vi "Autonomous Independent.vi"() -> ()   [LabVIEW 2012]
doc: "This VI is called when autonomous begins, and will automatically be terminated when autonomous ends. You can carry out timed or sensor driven robot movement independently without needing to return to the caller."
uses:
  <vilib>/Rock Robotics/WPI/Solenoid/WPI_SolenoidValue.ctl
  Robot Global Data.vi
  <vilib>/Rock Robotics/WPI/Compressor/WPI_CompressorGetSetRefNum.vi
  <vilib>/Rock Robotics/WPI/RobotDrive/WPI_RobotDriveGetSetRefNum.vi
  <vilib>/Rock Robotics/WPI/Solenoid/WPI_SolenoidSetEnum.vi
  <vilib>/Rock Robotics/WPI/RobotDrive/WPI_RobotDriveArcadeDrive_Standard(NoSaturation).vi
panel:
  out "Current Movement, for debugging":T1 {"Y Joystick Value" scale=1.0..-1.0; "X Joystick Value" scale=-1.0..1.0}
  in  "Array of robot movements":T2(array[cluster]) {"Y Joystick Value" scale=1.0..-1.0; "X Joystick Value" scale=-1.0..1.0}
  # "Be sure to right-click and choose Data Operations>>Make Current Value default if you want to save the array values with the VI"
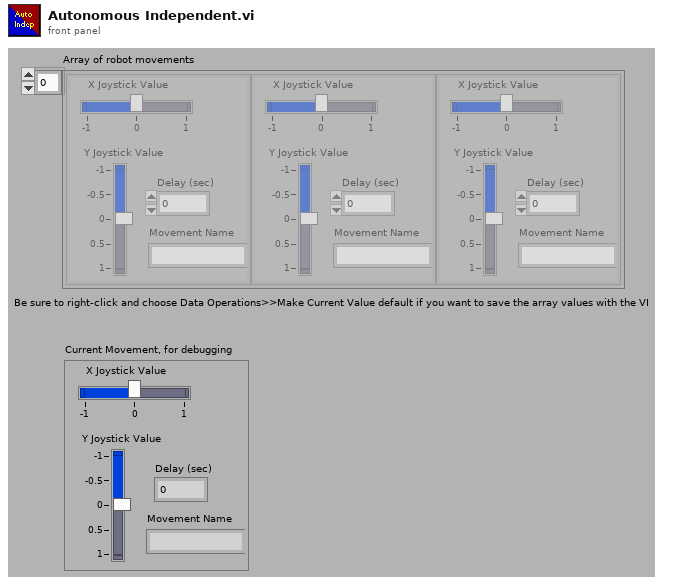
[diagram p1: front panel]
types:
  T1 = cluster{"X Joystick Value":dbl, "Y Joystick Value":dbl, "Delay (sec)":dbl, "Movement Name":string}
  T2 = cluster{"X Joystick Value":dbl, "Y Joystick Value":dbl, "Delay (sec)":dbl, "Movement Name":string}[]
  T3 = typedef "WPI_SolenoidDevRef.ctl" = cluster{"DevStatus":errorcluster, "Solenoid Module":T4, "Forward Solenoid Channel":T5, "Reverse Solenoid Channel":T5}
  T4 = typedef "FPGA_TypedefSolenoidModule.ctl" = enum16{"Solenoid Module 1", "Solenoid Module 2"}
  T5 = typedef "WPI_SolenoidChannel.ctl" = enum8{"Solenoid 1", "Solenoid 2", "Solenoid 3", "Solenoid 4", "Solenoid 5", "Solenoid 6", "Solenoid 7", "Solenoid 8", "Invalid"}
  T6 = typedef "WPI_MotorControlDeviceRef.ctl" = cluster{"DeviceStatus":errorcluster, "Type":enum16{"PWM", "CAN"}, "PWM":cluster{"Digital Module":T7, "PWM Channel":T8, "DeadBand":T9}, "CAN":cluster{"Device Number":u8, "Control Mode":T10, "Semaphore":T11, "Max Vout":dbl}, "Invert":bool, "TransformRef":T12, "InvTransformRef":T12}
  T7 = typedef "FPGA_TypedefDigitalModule.ctl" = enum16{"Digital Module 1", "Digital Module 2"}
  T8 = typedef "FPGA_DIOPWMChannel.ctl" = enum8{"PWM 1", "PWM 2", "PWM 3", "PWM 4", "PWM 5", "PWM 6", "PWM 7", "PWM 8", "PWM 9", "PWM 10", "Invalid"}
  T9 = typedef "WPI_PWMDeadband.ctl" = cluster{"Name":string, "maxPositivePwm":i32, "minPositivePwm":i32, "centerPwm":i32, "maxNegativePwm":i32, "minNegativePwm":i32, "angularRange":u16}
  T10 = typedef "WPI_CANJaguar_ControlMode.ctl" = enum8{"Percent VBus", "Current", "Speed", "Position", "Voltage"}
  T11 = typedef "Semaphore RefNum" = refnum<k1>
  T12 = typedef "WPI_PWMTransform_ConPane.ctl" = refnum<vi>
  T13 = typedef "WPI_DigitalInputDevRef.ctl" = cluster{"DevStatus":errorcluster, "DIO Channel":T14, "Digital Module":T7}
  T14 = typedef "FPGA_DIOChannel.ctl" = enum8{"DIO 1", "DIO 2", "DIO 3", "DIO 4", "DIO 5", "DIO 6", "DIO 7", "DIO 8", "DIO 9", "DIO 10", "DIO 11", "DIO 12", "DIO 13", "DIO 14", "Invalid"}
  T15 = typedef "WPI_SolenoidValue.ctl" = enum16{"Off", "On", "Forward", "Reverse"}
  T16 = typedef "WPI_RobotDriveDevRef.ctl" = cluster{"DevStatus":errorcluster, "Motors[]":T6[], "Square Inputs":bool, "Max Output":dbl, "Isochronous":bool}
  T17 = typedef "WPI_DigitalOutputDevRef.ctl" = cluster{"Digital Module":T7, "DIO Channel":T14, "DevStatus":errorcluster}
  T18 = typedef "WPI_CompressorDevRef.ctl" = cluster{"DevStatus":errorcluster, "DigitalInputDevRef":T13, "RelayDevRef":T19}
  T19 = typedef "WPI_RelayDevRef.ctl" = cluster{"DevStatus":errorcluster, "Relay Channel":T20, "Digital Module":T7, "Relay Direction":T21}
  T20 = typedef "FPGA_DIORelayChannel.ctl" = enum8{"Relay 1", "Relay 2", "Relay 3", "Relay 4", "Relay 5", "Relay 6", "Relay 7", "Relay 8", "Invalid"}
  T21 = typedef "WPI_RelayDirection.ctl" = enum16{"Both directions", "Forward only", "Reverse only"}
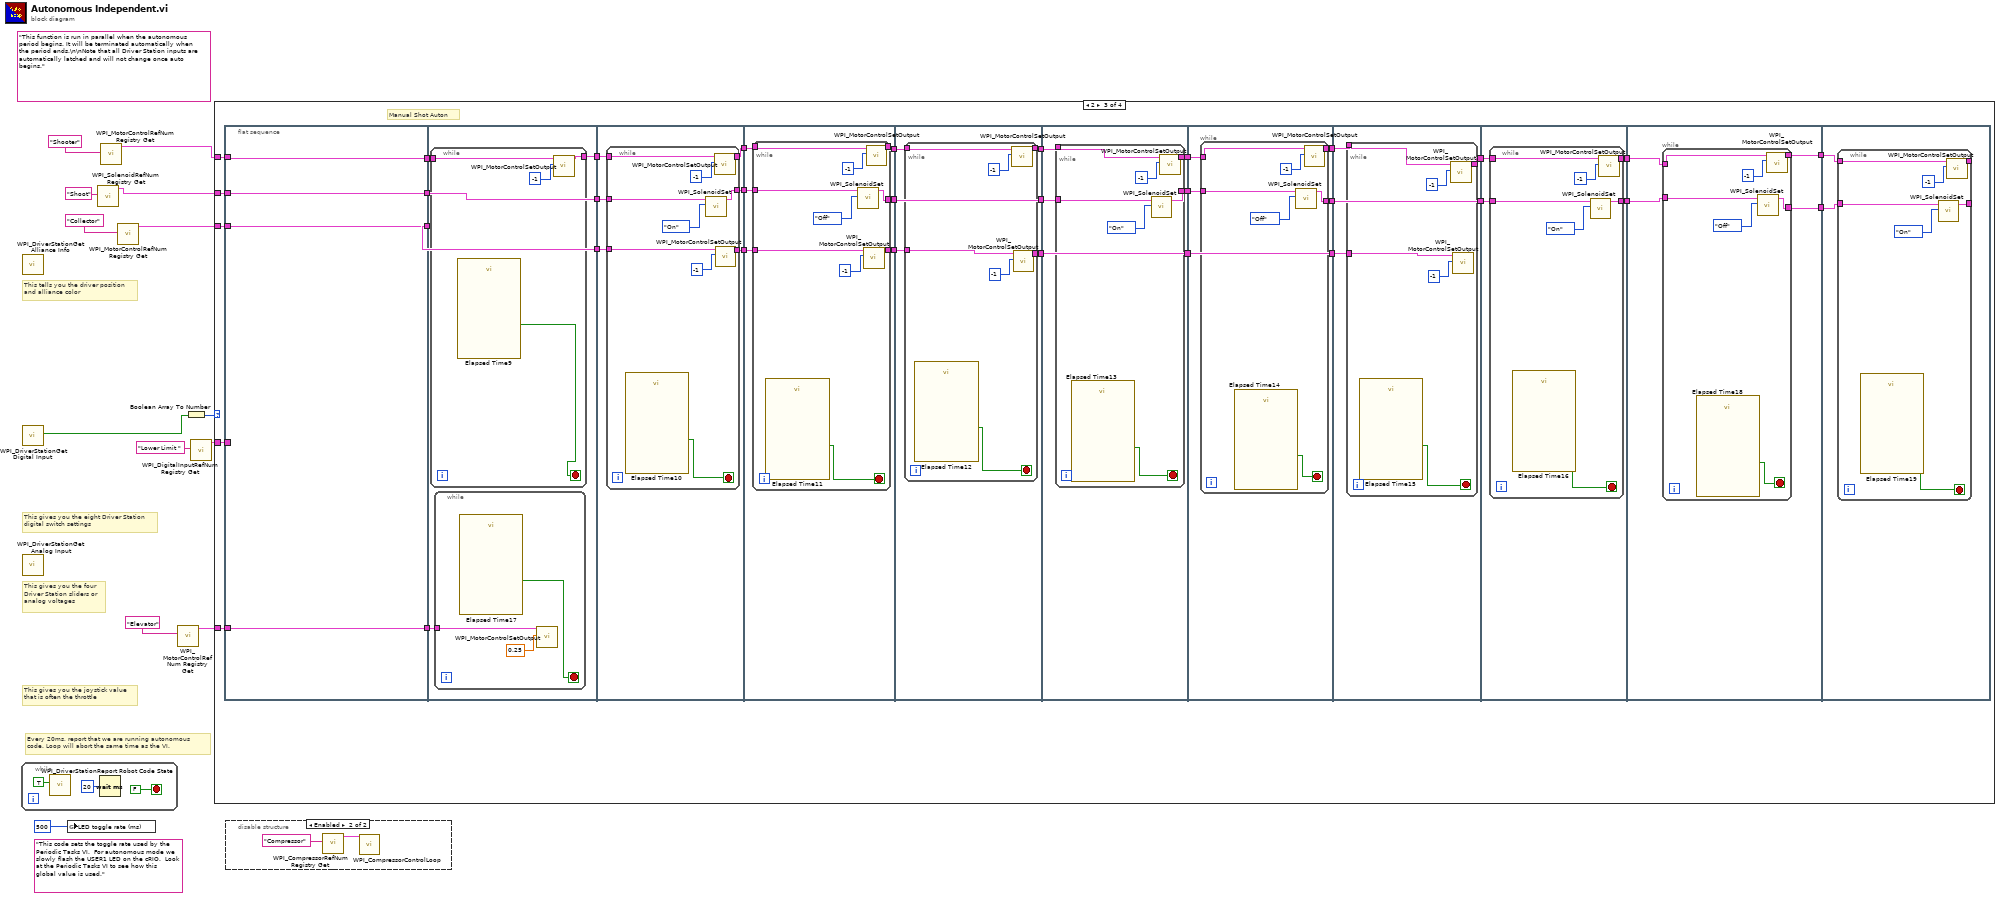
[diagram p0: block diagram]
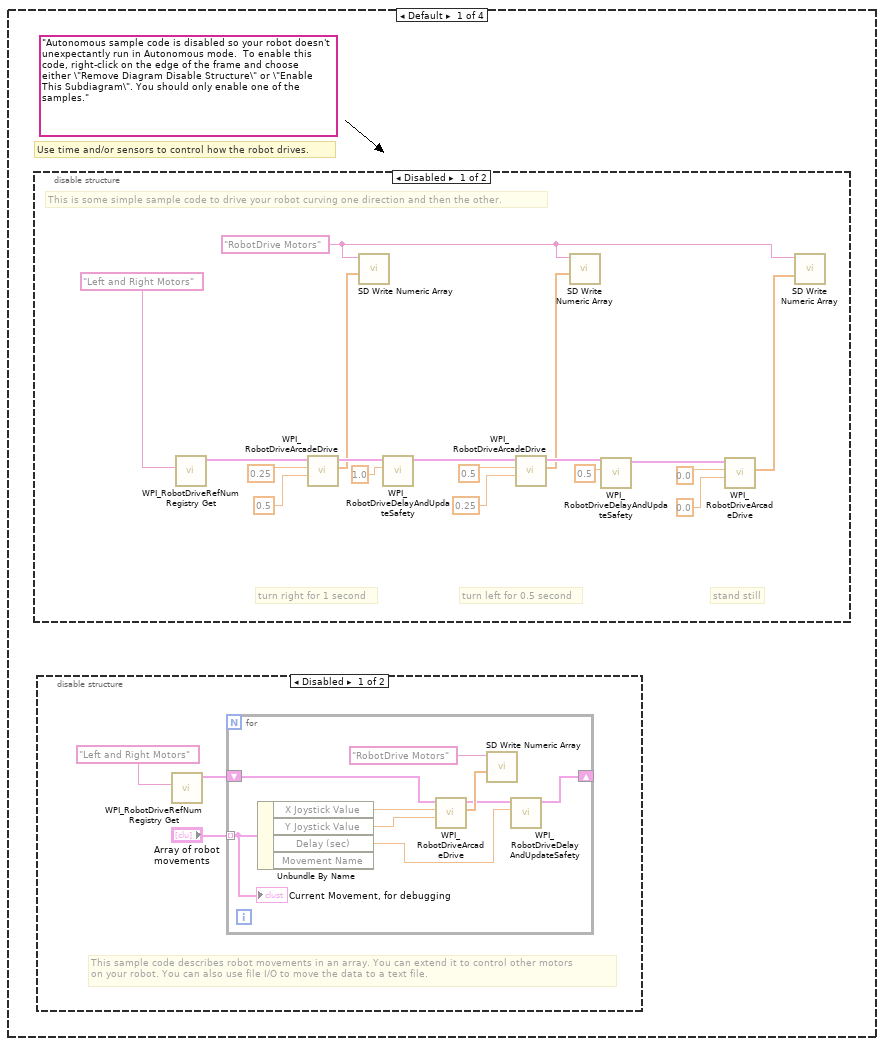
[diagram p3: hidden frame]
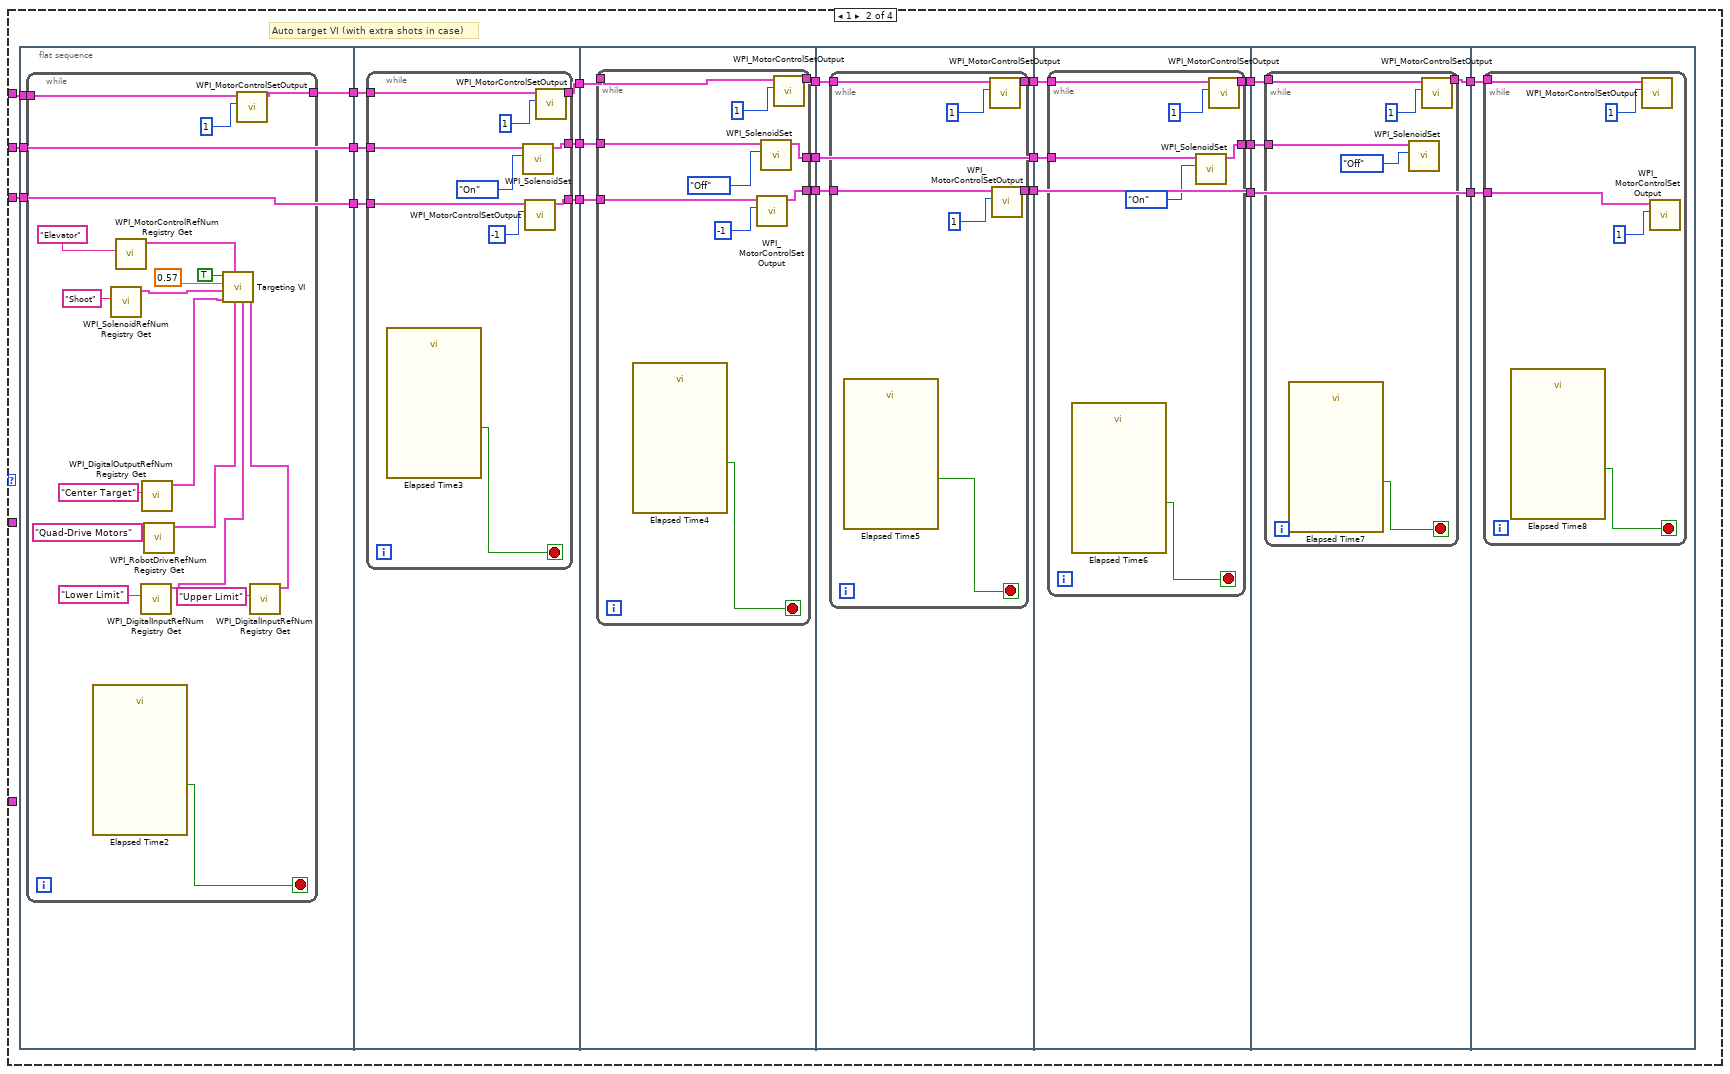
[diagram p6: hidden frame]
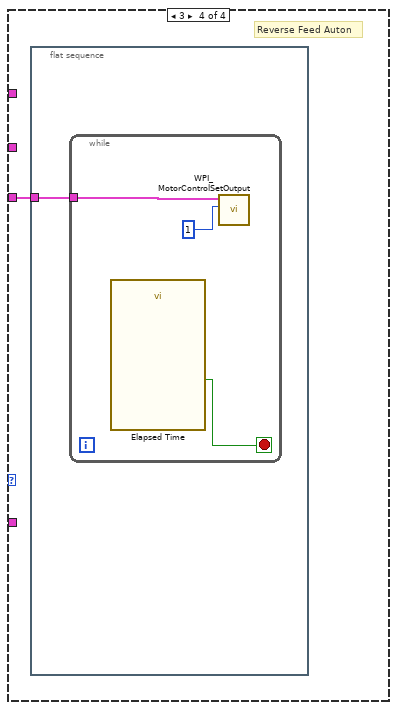
[diagram p7: hidden frame]
diagram:
  (unwired) "This code sets the toggle rate used by the Periodic Tasks VI.  For autonomous mode we slowly flash the USER1 LED on the cRIO.  Look at the Periodic Tasks VI to see how this global value is used."
  (unwired) "This function is run in parallel when the autonomous period begins. It will be terminated automatically when the period ends.\n\nNote that all Driver Station inputs are automatically latched and will not change once auto begins."
  # "Every 20ms, report that we are running autonomous\ncode. Loop will abort the same time as the VI."
  # "This gives you the joystick value\nthat is often the throttle"
  # "This tells you the driver position\nand alliance color"
  # "This gives you the eight Driver Station\ndigital switch settings"
  # "This gives you the four\nDriver Station sliders or\nanalog voltages"
  n1 = while {
    stop <- FALSE stop-if-true
    n2 = call <vilib>:"WPI_DriverStationReport Robot Code State.vi"("Autonomous"=TRUE) -> ()  [unwired: 10 in, 1 out]
    n3 = Wait (ms)(milliseconds to wait=u32 20) -> ()  [unwired: 1 out]
  }
  n4 = call <vilib>:"WPI_DriverStationGet Alliance Info.vi"() -> ()  [unwired: 12 out]
  n5 = call <vilib>:"WPI_DriverStationGet Digital Input.vi"() -> ("Driver Station Digital Input (1-8)"=w12:bool[])  [unwired: 11 out]
  n6 = call <vilib>:"WPI_DriverStationGet Analog Input.vi"() -> ()  [unwired: 12 out]
  n7 = global write "Robot Global Data.vi" "LED toggle rate (ms)"(u32 500 ("LED ms toggle rate")) -> ()
  n8 = call <vilib>:"WPI_SolenoidRefNum Registry Get.vi"("refnum name"="Shoot") -> ("SolenoidDevRef"=w8:T3)  [unwired: 9 in, 1 out]
  n9 = call <vilib>:"WPI_MotorControlRefNum Registry Get.vi"("refnum name"="Shooter") -> ("MotorControlDevRef"=w3:T6)  [unwired: 9 in, 1 out]
  n10 = call <vilib>:"WPI_MotorControlRefNum Registry Get.vi"("refnum name"="Collector") -> ("MotorControlDevRef"=w6:T6)  [unwired: 9 in, 1 out]
  n11 = call <vilib>:"WPI_MotorControlRefNum Registry Get.vi"("refnum name"="Elevator") -> ("MotorControlDevRef"=w4:T6)  [unwired: 9 in, 1 out]
  n12 = Boolean Array To Number(Boolean array=w12) -> (number=w11:u32)
  n13 = call <vilib>:"WPI_DigitalInputRefNum Registry Get.vi"("refnum name"="Lower Limit ") -> ("DigitalInputDevRef"=w2:T13)  [unwired: 9 in, 1 out]
  n14 = case shown="2" w11 {
    tunnel: w8 -> [_ w59 w185 _]
    tunnel: w6 -> [_ w53 w173 w319]
    tunnel: w4 -> [_ _ w171 _]
    tunnel: w3 -> [_ w47 w168 _]
    tunnel: w2 -> [_ _ w167 _]
    frame Default {
      (unwired) "Autonomous sample code is disabled so your robot doesn't unexpectantly run in Autonomous mode.  To enable this code, right-click on the edge of the frame and choose either \"Remove Diagram Disable Structure\" or \"Enable This Subdiagram\". You should only enable one of the samples."
      # "Use time and/or sensors to control how the robot drives."
      n15 = disable-structure shown="Disabled" {
        frame Disabled {
          w17 = "RobotDrive Motors" ("Name")
          # "This is some simple sample code to drive your robot curving one direction and then the other."
          # "stand still"
          # "turn left for 0.5 second"
          # "turn right for 1 second"
          n16 = call <vilib>:"WPI_RobotDriveRefNum Registry Get.vi"("refnum name"="Left and Right Motors") -> ("RobotDriveDevRef"=w21:T16)  [unwired: 1 in, 9 out]
          n17 = call-poly <vilib>:"WPI_RobotDriveArcadeDrive.vi"("Y axis value"=0.5 ("X axis value"), "X axis value"=0.25, "RobotDriveDevRef"=w21) -> ("Motor Values"=w20:dbl[], "RobotDriveDevRef"=w28:T16)  [unwired: 1 in, 6 out]
          n18 = call <vilib>:"SD Write Numeric Array.vi"("Numeric Array"=w20, "Name"=w17) -> ()  [unwired: 8 in, 2 out]
          n19 = call <vilib>:"WPI_RobotDriveDelayAndUpdateSafety.vi"("Delay (s)"=1.0, "RobotDriveDevRef"=w28) -> ("RobotDriveDevRef 2"=w27:T16)  [unwired: 8 in, 1 out]
          n20 = call-poly <vilib>:"WPI_RobotDriveArcadeDrive.vi"("Y axis value"=0.25 ("X axis value"), "X axis value"=0.5, "RobotDriveDevRef"=w27) -> ("Motor Values"=w19:dbl[], "RobotDriveDevRef"=w26:T16)  [unwired: 1 in, 6 out]
          n21 = call <vilib>:"SD Write Numeric Array.vi"("Numeric Array"=w19, "Name"=w17) -> ()  [unwired: 8 in, 2 out]
          n22 = call <vilib>:"WPI_RobotDriveDelayAndUpdateSafety.vi"("Delay (s)"=0.5, "RobotDriveDevRef"=w26) -> ("RobotDriveDevRef 2"=w25:T16)  [unwired: 8 in, 1 out]
          n23 = call-poly <vilib>:"WPI_RobotDriveArcadeDrive.vi"("Y axis value"=0.0 ("X axis value"), "X axis value"=0.0, "RobotDriveDevRef"=w25) -> ("Motor Values"=w18:dbl[])  [unwired: 1 in, 7 out]
          n24 = call <vilib>:"SD Write Numeric Array.vi"("Numeric Array"=w18, "Name"=w17) -> ()  [unwired: 8 in, 2 out]
        }
        frame Enabled {
        }
      }
      n25 = disable-structure shown="Disabled" {
        frame Disabled {
          # "This sample code describes robot movements in an array. You can extend it to control other motors\non your robot. You can also use file I/O to move the data to a text file."
          n26 = call <vilib>:"WPI_RobotDriveRefNum Registry Get.vi"("refnum name"="Left and Right Motors") -> ("RobotDriveDevRef"=w36:T16)  [unwired: 1 in, 9 out]
          n27 = for {
            shift-right: [w42] -> _
            shift-left: w36 -> [w43]
            tunnel: "Array of robot movements" -> [w38] mode=indexing
            n28 = Unbundle By Name(w38) -> ("X Joystick Value"=w41:dbl, "Y Joystick Value"=w40:dbl, "Delay (sec)"=w39:dbl)  [unwired: 1 out]
            n29 = call-poly <vilib>:"WPI_RobotDriveArcadeDrive.vi"("Y axis value"=w40, "X axis value"=w41, "RobotDriveDevRef"=w43) -> ("Motor Values"=w45:dbl[], "RobotDriveDevRef"=w44:T16)  [unwired: 1 in, 6 out]
            n30 = call <vilib>:"SD Write Numeric Array.vi"("Numeric Array"=w45, "Name"="RobotDrive Motors") -> ()  [unwired: 8 in, 2 out]
            n31 = call <vilib>:"WPI_RobotDriveDelayAndUpdateSafety.vi"("Delay (s)"=w39, "RobotDriveDevRef"=w44) -> ("RobotDriveDevRef 2"=w42:T16)  [unwired: 8 in, 1 out]
            "Current Movement, for debugging" <- w38
          }
        }
        frame Enabled {
        }
      }
    }
    frame 1 {
      # "Auto target VI (with extra shots in case)"
      n32 = flat-sequence {
        tunnel: [w70] -> w66
        tunnel: [w69] -> w60
        tunnel: w59 -> [w69]
        tunnel: [w68] -> w54
        tunnel: w53 -> [w68]
        tunnel: w47 -> [w67]
        tunnel: w66 -> [w93]
        tunnel: [w92] -> w65
        tunnel: w60 -> [w91]
        tunnel: [w90] -> w58
        tunnel: w54 -> [w89]
        tunnel: [w88] -> w52
        tunnel: w65 -> [w109]
        tunnel: [w108] -> w64
        tunnel: w58 -> [w107]
        tunnel: [w106] -> w57
        tunnel: w52 -> [w105]
        tunnel: [w104] -> w51
        tunnel: w64 -> [w124]
        tunnel: [w123] -> w63
        tunnel: w57 -> [w122]
        tunnel: [w122] -> w56
        tunnel: w51 -> [w121]
        tunnel: [w120] -> w48
        tunnel: w63 -> [w136]
        tunnel: [w135] -> w62
        tunnel: w56 -> [w134]
        tunnel: [w133] -> w55
        tunnel: [w132] -> w49
        tunnel: w48 -> [w132]
        tunnel: w62 -> [w147]
        tunnel: [w146] -> w61
        tunnel: w55 -> [w145]
        tunnel: [w144] -> w50
        tunnel: w49 -> [w144]
        tunnel: w61 -> [w155]
        tunnel: w50 -> [w154]
        frame #0 {
          n33 = while {
            tunnel: [w73] -> w70
            tunnel: w67 -> [w71]
            stop <- w72 stop-if-true
            (unwired) "Quad-Drive Motors" ("refnum name")
            n34 = call "Elapsed Time2"() -> ("Time has Elapsed"=w72:bool)  [unwired: 12 in, 7 out]
            n35 = call <vilib>:"WPI_SolenoidRefNum Registry Get.vi"("refnum name"="Shoot") -> ("SolenoidDevRef"=w81:T3)  [unwired: 9 in, 1 out]
            n36 = call <vilib>:"WPI_MotorControlRefNum Registry Get.vi"("refnum name"="Elevator") -> ("MotorControlDevRef"=w84:T6)  [unwired: 9 in, 1 out]
            n37 = call <vilib>:"WPI_DigitalInputRefNum Registry Get.vi"("refnum name"="Lower Limit") -> ("DigitalInputDevRef"=w75:T13)  [unwired: 9 in, 1 out]
            n38 = call <vilib>:"WPI_DigitalOutputRefNum Registry Get.vi"("refnum name"="Center Target") -> ("DigitalOutputDevRef"=w79:T17)  [unwired: 9 in, 1 out]
            n39 = call <vilib>:"WPI_RobotDriveRefNum Registry Get.vi"() -> ("RobotDriveDevRef"=w78:T16)  [unwired: 2 in, 9 out]
            n40 = call <vilib>:"WPI_MotorControlSetOutput.vi"("Output"=1, "MotorControlDevRef"=w71) -> ("MotorControlDevRef"=w73:T6)  [unwired: 7 in, 2 out]
            n41 = call <vilib>:"WPI_DigitalInputRefNum Registry Get.vi"("refnum name"="Upper Limit") -> ("DigitalInputDevRef"=w74:T13)  [unwired: 9 in, 1 out]
            n42 = call "Targeting VI.vi"("Upper Limit"=w74, "Lower Limit"=w75, "RobotDriveDevRef"=w78, "Elevator Control"=w84, "DO 14 LED"=w79, "Shoot"=w81, "slow turn"=0.57, "Aim Button"=TRUE) -> ()  [unwired: 4 in]
          }
        }
        frame #1 {
          n43 = while {
            tunnel: w93 -> [w100]
            tunnel: [w99] -> w92
            tunnel: w91 -> [w98]
            tunnel: [w97] -> w90
            tunnel: w89 -> [w96]
            tunnel: [w95] -> w88
            stop <- w94 stop-if-true
            n44 = call "Elapsed Time3"() -> ("Time has Elapsed"=w94:bool)  [unwired: 12 in, 7 out]
            n45 = call-poly <vilib>:"WPI_SolenoidSet.vi"("Value"=WPI_SolenoidValue."On", "SolenoidDevRef"=w98) -> ("SolenoidDevRef"=w97:T3)  [unwired: 8 in, 1 out]
            n46 = call <vilib>:"WPI_MotorControlSetOutput.vi"("Output"=-1, "MotorControlDevRef"=w96) -> ("MotorControlDevRef"=w95:T6)  [unwired: 7 in, 2 out]
            n47 = call <vilib>:"WPI_MotorControlSetOutput.vi"("Output"=1, "MotorControlDevRef"=w100) -> ("MotorControlDevRef"=w99:T6)  [unwired: 7 in, 2 out]
          }
        }
        frame #2 {
          n48 = while {
            tunnel: w109 -> [w116]
            tunnel: [w115] -> w108
            tunnel: w107 -> [w114]
            tunnel: [w113] -> w106
            tunnel: w105 -> [w112]
            tunnel: [w111] -> w104
            stop <- w110 stop-if-true
            n49 = call "Elapsed Time4"() -> ("Time has Elapsed"=w110:bool)  [unwired: 12 in, 7 out]
            n50 = call <vilib>:"WPI_MotorControlSetOutput.vi"("Output"=-1, "MotorControlDevRef"=w112) -> ("MotorControlDevRef"=w111:T6)  [unwired: 7 in, 2 out]
            n51 = call-poly <vilib>:"WPI_SolenoidSet.vi"("Value"=WPI_SolenoidValue."Off", "SolenoidDevRef"=w114) -> ("SolenoidDevRef"=w113:T3)  [unwired: 8 in, 1 out]
            n52 = call <vilib>:"WPI_MotorControlSetOutput.vi"("Output"=1, "MotorControlDevRef"=w116) -> ("MotorControlDevRef"=w115:T6)  [unwired: 7 in, 2 out]
          }
        }
        frame #3 {
          n53 = while {
            tunnel: w124 -> [w129]
            tunnel: [w128] -> w123
            tunnel: w121 -> [w127]
            tunnel: [w126] -> w120
            stop <- w125 stop-if-true
            n54 = call "Elapsed Time5"() -> ("Time has Elapsed"=w125:bool)  [unwired: 12 in, 7 out]
            n55 = call <vilib>:"WPI_MotorControlSetOutput.vi"("Output"=1, "MotorControlDevRef"=w129) -> ("MotorControlDevRef"=w128:T6)  [unwired: 7 in, 2 out]
            n56 = call <vilib>:"WPI_MotorControlSetOutput.vi"("Output"=1, "MotorControlDevRef"=w127) -> ("MotorControlDevRef"=w126:T6)  [unwired: 7 in, 2 out]
          }
        }
        frame #4 {
          n57 = while {
            tunnel: w136 -> [w141]
            tunnel: [w140] -> w135
            tunnel: w134 -> [w139]
            tunnel: [w138] -> w133
            stop <- w137 stop-if-true
            n58 = call "Elapsed Time6"() -> ("Time has Elapsed"=w137:bool)  [unwired: 12 in, 7 out]
            n59 = call-poly <vilib>:"WPI_SolenoidSet.vi"("Value"=WPI_SolenoidValue."On", "SolenoidDevRef"=w139) -> ("SolenoidDevRef"=w138:T3)  [unwired: 8 in, 1 out]
            n60 = call <vilib>:"WPI_MotorControlSetOutput.vi"("Output"=1, "MotorControlDevRef"=w141) -> ("MotorControlDevRef"=w140:T6)  [unwired: 7 in, 2 out]
          }
        }
        frame #5 {
          n61 = while {
            tunnel: w147 -> [w151]
            tunnel: [w150] -> w146
            tunnel: w145 -> [w149]
            stop <- w148 stop-if-true
            n62 = call "Elapsed Time7"() -> ("Time has Elapsed"=w148:bool)  [unwired: 12 in, 7 out]
            n63 = call-poly <vilib>:"WPI_SolenoidSet.vi"("Value"=WPI_SolenoidValue."Off", "SolenoidDevRef"=w149) -> ()  [unwired: 8 in, 2 out]
            n64 = call <vilib>:"WPI_MotorControlSetOutput.vi"("Output"=1, "MotorControlDevRef"=w151) -> ("MotorControlDevRef"=w150:T6)  [unwired: 7 in, 2 out]
          }
        }
        frame #6 {
          n65 = while {
            tunnel: w155 -> [w158]
            tunnel: w154 -> [w157]
            stop <- w156 stop-if-true
            n66 = call "Elapsed Time8"() -> ("Time has Elapsed"=w156:bool)  [unwired: 12 in, 7 out]
            n67 = call <vilib>:"WPI_MotorControlSetOutput.vi"("Output"=1, "MotorControlDevRef"=w158) -> ()  [unwired: 7 in, 3 out]
            n68 = call <vilib>:"WPI_MotorControlSetOutput.vi"("Output"=1, "MotorControlDevRef"=w157) -> ()  [unwired: 7 in, 3 out]
          }
        }
      }
    }
    frame 2 {
      # "Manual Shot Auton"
      n69 = flat-sequence {
        tunnel: w171 -> [w196]
        tunnel: w173 -> [w194]
        tunnel: w185 -> [w197]
        tunnel: [w197] -> w170
        tunnel: [w196] -> w169
        tunnel: w168 -> [w195]
        tunnel: w167 -> [_]
        tunnel: [w195] -> w166
        tunnel: [w194] -> w165
        tunnel: [w202] -> w193
        tunnel: [w201] -> w186
        tunnel: [w200] -> w172
        tunnel: w170 -> [w201]
        tunnel: w169 -> [w199]
        tunnel: w166 -> [w198]
        tunnel: w165 -> [w200]
        tunnel: w193 -> [w215]
        tunnel: [w214] -> w192
        tunnel: w186 -> [w213]
        tunnel: [w212] -> w184
        tunnel: [w211] -> w174
        tunnel: w172 -> [w210]
        tunnel: w192 -> [w231]
        tunnel: [w230] -> w191
        tunnel: w184 -> [w229]
        tunnel: [w228] -> w182
        tunnel: [w227] -> w175
        tunnel: w174 -> [w226]
        tunnel: w191 -> [w246]
        tunnel: [w245] -> w190
        tunnel: [w244] -> w183
        tunnel: w182 -> [w244]
        tunnel: [w243] -> w178
        tunnel: w175 -> [w242]
        tunnel: w190 -> [w258]
        tunnel: [w257] -> w189
        tunnel: w183 -> [w256]
        tunnel: [w255] -> w181
        tunnel: w178 -> [w254]
        tunnel: [w254] -> w177
        tunnel: w189 -> [w270]
        tunnel: [w269] -> w188
        tunnel: w181 -> [w268]
        tunnel: [w267] -> w179
        tunnel: w177 -> [w266]
        tunnel: [w266] -> w176
        tunnel: w188 -> [w281]
        tunnel: [w280] -> w187
        tunnel: [w279] -> w180
        tunnel: w179 -> [w279]
        tunnel: w176 -> [w278]
        tunnel: w187 -> [w291]
        tunnel: w180 -> [w290]
        tunnel: [w289] -> w164
        tunnel: [w288] -> w163
        tunnel: w164 -> [w302]
        tunnel: w163 -> [w301]
        tunnel: [w300] -> w162
        tunnel: [w299] -> w161
        tunnel: w162 -> [w311]
        tunnel: w161 -> [w310]
        frame #0 {
        }
        frame #1 {
          n70 = while {
            tunnel: [w208] -> w202
            tunnel: w198 -> [w206]
            stop <- w207 stop-if-true
            n71 = call "Elapsed Time9"() -> ("Time has Elapsed"=w207:bool)  [unwired: 12 in, 7 out]
            n72 = call <vilib>:"WPI_MotorControlSetOutput.vi"("Output"=-1, "MotorControlDevRef"=w206) -> ("MotorControlDevRef"=w208:T6)  [unwired: 7 in, 2 out]
          }
          n73 = while {
            tunnel: w199 -> [w204]
            stop <- w203 stop-if-true
            n74 = call "Elapsed Time17"() -> ("Time has Elapsed"=w203:bool)  [unwired: 12 in, 7 out]
            n75 = call <vilib>:"WPI_MotorControlSetOutput.vi"("Output"=0.25, "MotorControlDevRef"=w204) -> ()  [unwired: 7 in, 3 out]
          }
        }
        frame #2 {
          n76 = while {
            tunnel: w215 -> [w222]
            tunnel: [w221] -> w214
            tunnel: w213 -> [w220]
            tunnel: [w219] -> w212
            tunnel: [w218] -> w211
            tunnel: w210 -> [w217]
            stop <- w216 stop-if-true
            n77 = call "Elapsed Time10"() -> ("Time has Elapsed"=w216:bool)  [unwired: 12 in, 7 out]
            n78 = call-poly <vilib>:"WPI_SolenoidSet.vi"("Value"=WPI_SolenoidValue."On", "SolenoidDevRef"=w220) -> ("SolenoidDevRef"=w219:T3)  [unwired: 8 in, 1 out]
            n79 = call <vilib>:"WPI_MotorControlSetOutput.vi"("Output"=-1, "MotorControlDevRef"=w222) -> ("MotorControlDevRef"=w221:T6)  [unwired: 7 in, 2 out]
            n80 = call <vilib>:"WPI_MotorControlSetOutput.vi"("Output"=-1, "MotorControlDevRef"=w217) -> ("MotorControlDevRef"=w218:T6)  [unwired: 7 in, 2 out]
          }
        }
        frame #3 {
          n81 = while {
            tunnel: w231 -> [w238]
            tunnel: [w237] -> w230
            tunnel: w229 -> [w236]
            tunnel: [w235] -> w228
            tunnel: [w234] -> w227
            tunnel: w226 -> [w233]
            stop <- w232 stop-if-true
            n82 = call "Elapsed Time11"() -> ("Time has Elapsed"=w232:bool)  [unwired: 12 in, 7 out]
            n83 = call-poly <vilib>:"WPI_SolenoidSet.vi"("Value"=WPI_SolenoidValue."Off", "SolenoidDevRef"=w236) -> ("SolenoidDevRef"=w235:T3)  [unwired: 8 in, 1 out]
            n84 = call <vilib>:"WPI_MotorControlSetOutput.vi"("Output"=-1, "MotorControlDevRef"=w233) -> ("MotorControlDevRef"=w234:T6)  [unwired: 7 in, 2 out]
            n85 = call <vilib>:"WPI_MotorControlSetOutput.vi"("Output"=-1, "MotorControlDevRef"=w238) -> ("MotorControlDevRef"=w237:T6)  [unwired: 7 in, 2 out]
          }
        }
        frame #4 {
          n86 = while {
            tunnel: w246 -> [w251]
            tunnel: [w250] -> w245
            tunnel: [w249] -> w243
            tunnel: w242 -> [w247]
            stop <- w248 stop-if-true
            n87 = call "Elapsed Time12"() -> ("Time has Elapsed"=w248:bool)  [unwired: 12 in, 7 out]
            n88 = call <vilib>:"WPI_MotorControlSetOutput.vi"("Output"=-1, "MotorControlDevRef"=w251) -> ("MotorControlDevRef"=w250:T6)  [unwired: 7 in, 2 out]
            n89 = call <vilib>:"WPI_MotorControlSetOutput.vi"("Output"=-1, "MotorControlDevRef"=w247) -> ("MotorControlDevRef"=w249:T6)  [unwired: 7 in, 2 out]
          }
        }
        frame #5 {
          n90 = while {
            tunnel: w258 -> [w263]
            tunnel: [w262] -> w257
            tunnel: w256 -> [w261]
            tunnel: [w260] -> w255
            stop <- w259 stop-if-true
            n91 = call "Elapsed Time13"() -> ("Time has Elapsed"=w259:bool)  [unwired: 12 in, 7 out]
            n92 = call-poly <vilib>:"WPI_SolenoidSet.vi"("Value"=WPI_SolenoidValue."On", "SolenoidDevRef"=w261) -> ("SolenoidDevRef"=w260:T3)  [unwired: 8 in, 1 out]
            n93 = call <vilib>:"WPI_MotorControlSetOutput.vi"("Output"=-1, "MotorControlDevRef"=w263) -> ("MotorControlDevRef"=w262:T6)  [unwired: 7 in, 2 out]
          }
        }
        frame #6 {
          n94 = while {
            tunnel: w270 -> [w275]
            tunnel: [w274] -> w269
            tunnel: w268 -> [w273]
            tunnel: [w272] -> w267
            stop <- w271 stop-if-true
            n95 = call "Elapsed Time14"() -> ("Time has Elapsed"=w271:bool)  [unwired: 12 in, 7 out]
            n96 = call-poly <vilib>:"WPI_SolenoidSet.vi"("Value"=WPI_SolenoidValue."Off", "SolenoidDevRef"=w273) -> ("SolenoidDevRef"=w272:T3)  [unwired: 8 in, 1 out]
            n97 = call <vilib>:"WPI_MotorControlSetOutput.vi"("Output"=-1, "MotorControlDevRef"=w275) -> ("MotorControlDevRef"=w274:T6)  [unwired: 7 in, 2 out]
          }
        }
        frame #7 {
          n98 = while {
            tunnel: w281 -> [w285]
            tunnel: [w284] -> w280
            tunnel: w278 -> [w283]
            stop <- w282 stop-if-true
            n99 = call "Elapsed Time15"() -> ("Time has Elapsed"=w282:bool)  [unwired: 12 in, 7 out]
            n100 = call <vilib>:"WPI_MotorControlSetOutput.vi"("Output"=-1, "MotorControlDevRef"=w285) -> ("MotorControlDevRef"=w284:T6)  [unwired: 7 in, 2 out]
            n101 = call <vilib>:"WPI_MotorControlSetOutput.vi"("Output"=-1, "MotorControlDevRef"=w283) -> ()  [unwired: 7 in, 3 out]
          }
        }
        frame #8 {
          n102 = while {
            tunnel: w291 -> [w296]
            tunnel: w290 -> [w295]
            tunnel: [w293] -> w289
            tunnel: [w292] -> w288
            stop <- w294 stop-if-true
            n103 = call "Elapsed Time16"() -> ("Time has Elapsed"=w294:bool)  [unwired: 12 in, 7 out]
            n104 = call-poly <vilib>:"WPI_SolenoidSet.vi"("Value"=WPI_SolenoidValue."On", "SolenoidDevRef"=w295) -> ("SolenoidDevRef"=w293:T3)  [unwired: 8 in, 1 out]
            n105 = call <vilib>:"WPI_MotorControlSetOutput.vi"("Output"=-1, "MotorControlDevRef"=w296) -> ("MotorControlDevRef"=w292:T6)  [unwired: 7 in, 2 out]
          }
        }
        frame #9 {
          n106 = while {
            tunnel: w301 -> [w307]
            tunnel: [w306] -> w299
            tunnel: w302 -> [w305]
            tunnel: [w304] -> w300
            stop <- w303 stop-if-true
            n107 = call "Elapsed Time18"() -> ("Time has Elapsed"=w303:bool)  [unwired: 12 in, 7 out]
            n108 = call-poly <vilib>:"WPI_SolenoidSet.vi"("Value"=WPI_SolenoidValue."Off", "SolenoidDevRef"=w305) -> ("SolenoidDevRef"=w304:T3)  [unwired: 8 in, 1 out]
            n109 = call <vilib>:"WPI_MotorControlSetOutput.vi"("Output"=-1, "MotorControlDevRef"=w307) -> ("MotorControlDevRef"=w306:T6)  [unwired: 7 in, 2 out]
          }
        }
        frame #10 {
          n110 = while {
            tunnel: w310 -> [w316]
            tunnel: w311 -> [w315]
            tunnel: [w313] -> _
            tunnel: [w312] -> _
            stop <- w314 stop-if-true
            n111 = call "Elapsed Time19"() -> ("Time has Elapsed"=w314:bool)  [unwired: 12 in, 7 out]
            n112 = call-poly <vilib>:"WPI_SolenoidSet.vi"("Value"=WPI_SolenoidValue."On", "SolenoidDevRef"=w315) -> ("SolenoidDevRef"=w313:T3)  [unwired: 8 in, 1 out]
            n113 = call <vilib>:"WPI_MotorControlSetOutput.vi"("Output"=-1, "MotorControlDevRef"=w316) -> ("MotorControlDevRef"=w312:T6)  [unwired: 7 in, 2 out]
          }
        }
      }
    }
    frame 3 {
      # "Reverse Feed Auton"
      n114 = flat-sequence {
        tunnel: w319 -> [w320]
        frame #0 {
          n115 = while {
            tunnel: w320 -> [w322]
            stop <- w321 stop-if-true
            n116 = call "Elapsed Time"() -> ("Time has Elapsed"=w321:bool)  [unwired: 12 in, 7 out]
            n117 = call <vilib>:"WPI_MotorControlSetOutput.vi"("Output"=1, "MotorControlDevRef"=w322) -> ()  [unwired: 7 in, 3 out]
          }
        }
      }
    }
  }
  n118 = disable-structure shown="Enabled" {
    frame Disabled {
    }
    frame Enabled {
      n119 = call <vilib>:"WPI_CompressorRefNum Registry Get.vi"("refnum name"="Compressor") -> ("CompressorDevRef"=w325:T18)  [unwired: 9 in, 1 out]
      n120 = call <vilib>:"WPI_CompressorControlLoop.vi"("CompressorDevRef"=w325) -> ()  [unwired: 11 in]
    }
  }
